vi "Read Measurement Data.vi"(8 "error in (no error)":errorcluster, 11 "Device ID (0)":i32) -> (0 "error out":errorcluster, 2 "Measure Data":T1[](array[typedef]) {"Judge Result" items=["HI"=1, "GO"=2, "LO"=4, "ALARM"=5]; "Data Info" items=["VALID", "ALARM", "WAIT"]}, 3 "Device ID out":i32)   [LabVIEW 2014, in "Keyence LJ-V7000.lvlib"]
doc: "This function gets the newest measurement results (measurement values and judgment results)."
uses:
  Keyence LJ-V7000.lvlib
  Clusters/Measure Data.ctl
  constant/Measure Data Info.ctl
  constant/Judge Result.ctl
  constant/Driver VI No.ctl
panel:
  # "(c) 2012 KEYENCE CORPORATION.  ALL RIGHTS RESERVED."
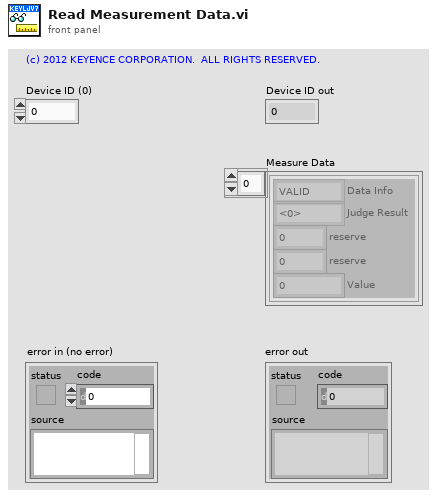
[diagram p1: front panel]
types:
  T1 = typedef "Keyence LJ-V7000.lvlib/Measure Data.ctl" = cluster{"Data Info":T2, "Judge Result":T3, "reserve":u8, "reserve":u8, "Value":sgl}
  T2 = typedef "Keyence LJ-V7000.lvlib/Measure Data Info.ctl" = u8
  T3 = typedef "Keyence LJ-V7000.lvlib/Judge Result.ctl" = u8
  T4 = typedef "Keyence LJ-V7000.lvlib/Driver VI No.ctl" = enum16{"Initialize", "Close", "Reboot Controller", "Return to Factory State", "Get System Error", "Clear System Error", "Trigger", "Start Batch Measurements", "Stop Batch Measurements", "Auto Zero", "Timing", "Reset", "Clear Memory", "Set Setting", "Get Setting", "Initialize Setting", "Reflect Setting", "Update Write Settings Area", "Check Status of Saving to Save Area", "Set Time", "Get Time", "Change Program", "Read Active Program Number", "Read Measurement Data", "Read Profiles(for High-Speed Mode)", "Read Batch Profiles(for High-Speed Mode)", "Read Profiles(for Advanced Mode)", "Read Batch Profiles(for Advanced Mode)", "Start Storage", "Stop Storage", "Read Storage Status", "Read Data Storage Data", "Read Profile Storage Data", "Read Batch Profile Storage Data", "Start High-Speed Data Communication", "Stop High-Speed Data Communication", "Read Profiles(for High-Speed Communication)"}
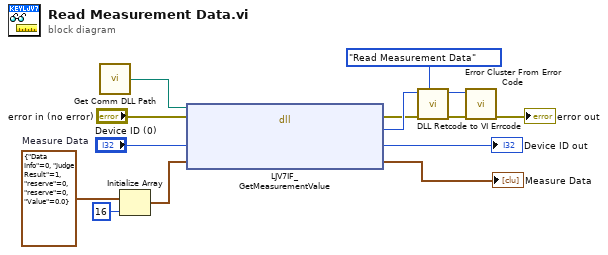
[diagram p0: block diagram]
diagram:
  w10 = T1 {"Data Info"=0, "Judge Result"=1, "reserve"=0, "reserve"=0, "Value"=0.0}  # Measure Data
  n1 = call "Get Comm DLL Path.vi"() -> ("Comm DLL Path"=w12:path)  [unwired: 1 in]
  n2 = Initialize Array(w10, 16 ("次元サイズ")) -> (w8:T1[])
  n3 = dll-call lib="C:/Program Files/National Instruments/LabVIEW 2011/instr.lib/Keyence LJ-V7000/LJV7_IF.*" fn="LJV7IF_GetMeasurementValue"(path in=w12, error in="error in (no error)", "lDeviceId"="Device ID (0)", "pMeasureData"=w8) -> (error out=w3:errorcluster, "lRetCode"=w4:i32, "lDeviceId"=→"Device ID out":i32, "pMeasureData"=→"Measure Data":T1[])  [unwired: 1 in, 1 out]
  n4 = call "DLL Retcode to VI Errcode.vi"("Driver VI No"=Driver_VI_No."Read Measurement Data", "error in (no error)"=w3, "DLL Return Code"=w4) -> ("error out"=w6:errorcluster, "VI Error Code"=w5:i32)  [unwired: 7 in]
  n5 = call <vilib>:"Error Cluster From Error Code.vi"("error in (no error)"=w6, "error code (0)"=w5) -> ("error out"=→"error out":errorcluster)  [unwired: 7 in]
